vi "TestOdometry.vi"() -> ()   [LabVIEW 2018]
panel:
  out "XY Graph":cluster{dbl[], dbl[]}(graph)
  in  "stop":bool
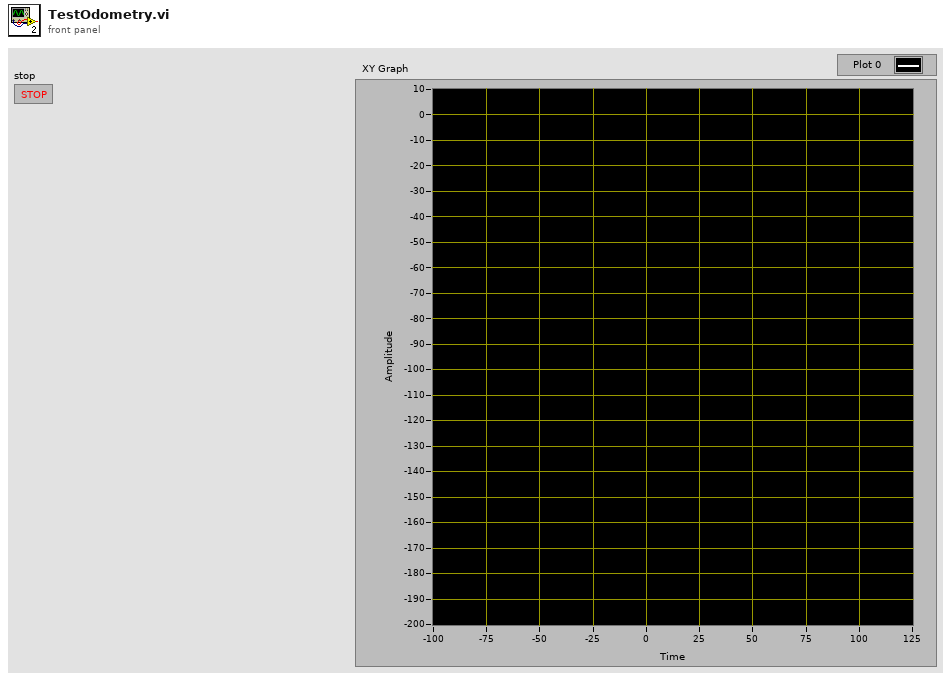
[diagram p1: front panel]
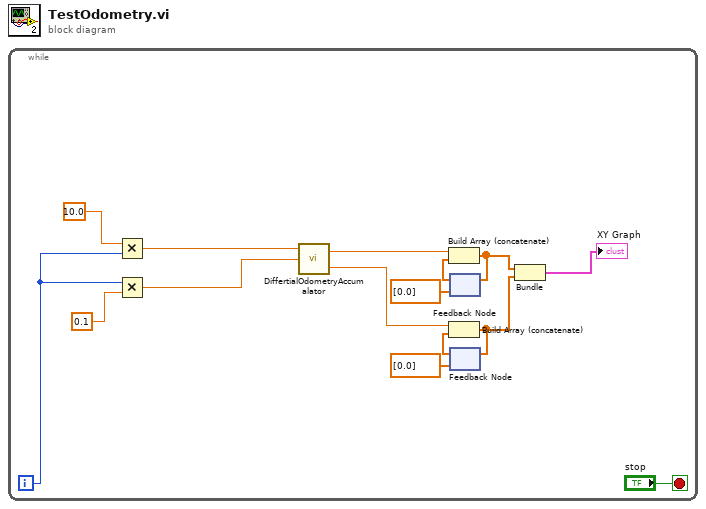
[diagram p0: block diagram]
diagram:
  n1 = while {
    i -> [w12]
    stop <- "stop" stop-if-true
    n2 = Multiply(x=10.0, y=w12) -> (x*y=w13:dbl)
    n3 = Multiply(x=w12, y=0.1) -> (x*y=w10:dbl)
    n4 = call "DiffertialOdometryAccumalator.vi"("Position"=w13, "Heading (rad)"=w10) -> ("X"=w9:dbl, "Y"=w4:dbl)  [unwired: 3 in]
    n5 = feedback #1(dbl[] [0.0]) -> (w8:dbl[])
    n6 = Build Array (concatenate)(w9, w8) -> (w3:dbl[])
    n7 = feedback-in #1(w3) -> ()
    n8 = feedback #2(dbl[] [0.0]) -> (w5:dbl[])
    n9 = Build Array (concatenate)(w4, w5) -> (w2:dbl[])
    n10 = feedback-in #2(w2) -> ()
    n11 = Bundle(w3, w2) -> (→"XY Graph":cluster{dbl[], dbl[]})  [unwired: 1 in]
  }
